vi "return_axis.vi"(7 "u(0)":sgl format="%#_13g", 8 "TsTicks":u32=1600, 10 "phony-enable":bool, 11 "FPGA I/O In":refnum<k21>="Mod1/AO0") -> (3 "finished":bool)   [LabVIEW 2017]
uses:
  <vilib>/rvi/Emulation/niFpgaGetClockAttributes.vi
  <vilib>/rvi/Emulation/niFpgaSctlEmulationGetInTimedLoop.vi
  <vilib>/rvi/Emulation/niFpgaEmulationReportErrorSimple.vi
  <vilib>/rvi/eio/common/nirviEmuTemplateMethod_errors.vi
  <vilib>/rvi/Emulation/niFpgaCriticalErrorInLSC.vi
  <vilib>/eio/EIONode/EIONode.xnode
panel:
  out "Ux":sgl
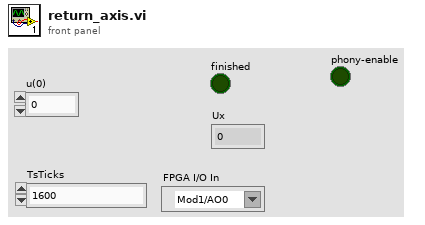
[diagram p1: front panel]
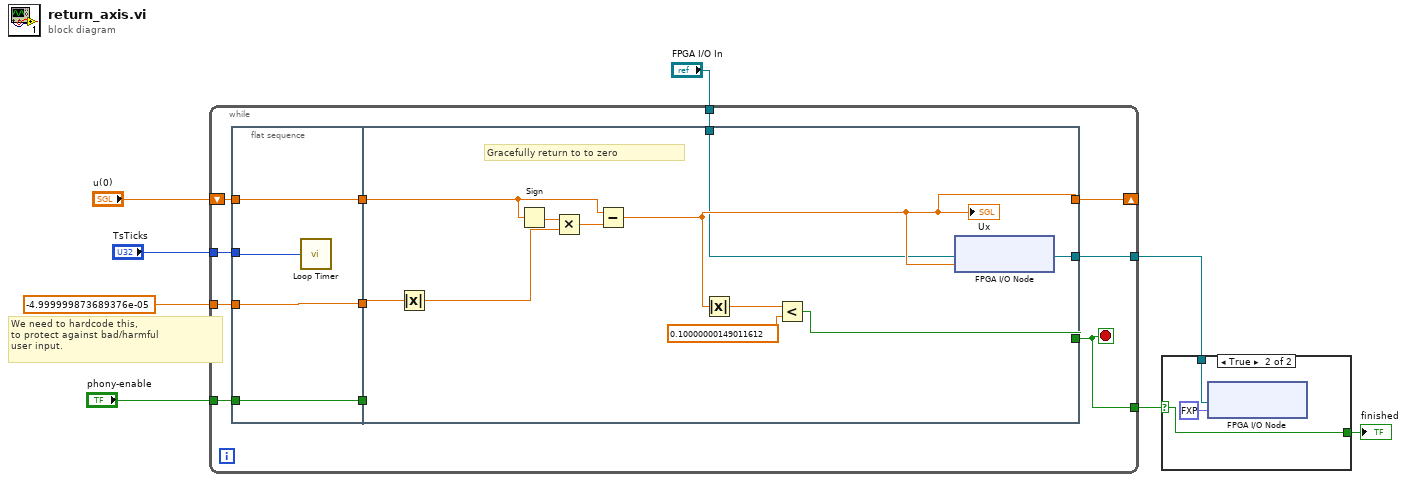
[diagram p0: block diagram]
diagram:
  # "We need to hardcode this,\nto protect against bad/harmful\nuser input."
  n1 = while {
    tunnel: sgl -5e-05 -> [w17]
    shift-right: [w16] -> _
    shift-left: "u(0)" -> [w15]
    tunnel: [w14] -> w7
    tunnel: "TsTicks" -> [w13]
    tunnel: "FPGA I/O In" -> [w12]
    tunnel: [w11] -> w3
    tunnel: "phony-enable" -> [w9]
    stop <- w14 stop-if-true
    n2 = flat-sequence {
      tunnel: [w23] -> w19
      tunnel: w15 -> [w23]
      tunnel: [w22] -> w18
      tunnel: w17 -> [w22]
      tunnel: w13 -> [w21]
      tunnel: [w20] -> w10
      tunnel: w9 -> [w20]
      tunnel: w19 -> [w31]
      tunnel: w18 -> [w29]
      tunnel: [w26] -> w14
      tunnel: [w30] -> w16
      tunnel: w12 -> [w25]
      tunnel: [w24] -> w11
      tunnel: w10 -> [_]
      frame #0 {
        n3 = call "Loop Timer"("Count(Ticks)"=w21) -> ()  [unwired: 1 out]
      }
      frame #1 {
        # "Gracefully return to to zero"
        n4 = Absolute Value(x=w29) -> (abs(x)=w28:sgl)
        n5 = Sign(1:w31) -> (0:w33:sgl)
        n6 = Multiply(x=w33, y=w28) -> (x*y=w34:sgl)
        n7 = Subtract(x=w31, y=w34) -> (x-y=w30:sgl)
        "Ux" <- w30
        n8 = Absolute Value(x=w30) -> (abs(x)=w32:sgl)
        n9 = Less?(x=w32, y=sgl 0.1) -> (x < y?=w26:bool)
        n10 = xnode "FPGA I/O Node"("I/O Item"=w30, "FPGA I/O In"=w25) -> ("FPGA I/O Out"=w24:refnum<k21>)
      }
    }
  }
  n11 = case shown="True" w7 {
    selector: w7 -> [w35 w36]
    tunnel: w3 -> [_ w38]
    tunnel: [w35 w36] -> w2
    frame False {
    }
    frame True {
      n12 = xnode "FPGA I/O Node"("I/O Item"=fxp<+/-,20,5> 0.0, "FPGA I/O In"=w38) -> ()  [unwired: 1 out]
    }
  }
  "finished" <- w2
